vi "ScanPositionRange.vi"(8 "Target position":dbl, 9 "Start position":dbl, 10 "Velocity":dbl, 11 "Connection Cluster in":T1) -> (1 "Peak detected?":bool, 2 "output cluster":cluster{dbl[], dbl[]}, 3 "Connection Cluster out":T1)   [LabVIEW 2013]
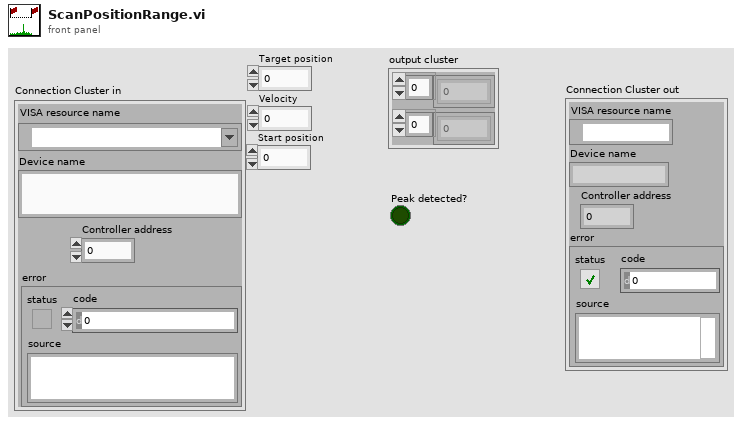
[diagram p1: front panel]
types:
  T1 = cluster{"VISA resource name":refnum<visa-resource-name>, "Device name":string, "Controller address":i32, "error":errorcluster}
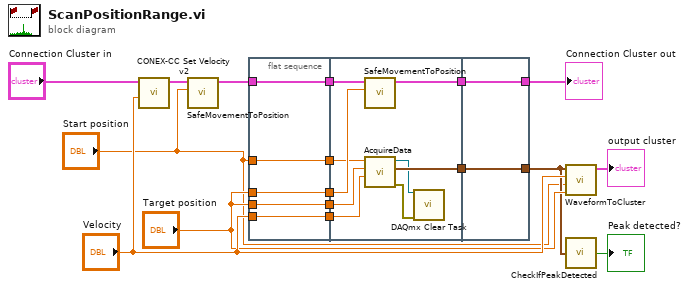
[diagram p0: block diagram]
diagram:
  n1 = call <userlib>:"CONEX-CC Set Velocity v2.vi"("Velocity"="Velocity", "Connection Cluster in"="Connection Cluster in") -> ("Connection Cluster out"=w14:T1)  [unwired: 9 in]
  n2 = call "SafeMovementToPosition.vi"("Target position"="Start position", "Connection Cluster in"=w14) -> ("Connection Cluster out"=w17:T1)  [unwired: 9 in]
  n3 = flat-sequence {
    tunnel: "Velocity" -> [w18]
    tunnel: "Target position" -> [w19]
    tunnel: "Start position" -> [w20]
    tunnel: "Target position" -> [w21]
    tunnel: w17 -> [w22]
    tunnel: [w22] -> w11
    tunnel: [w21] -> w10
    tunnel: [w20] -> w9
    tunnel: [w19] -> w8
    tunnel: [w18] -> w7
    tunnel: w11 -> [w31]
    tunnel: w10 -> [w28]
    tunnel: w9 -> [w27]
    tunnel: w8 -> [w26]
    tunnel: w7 -> [w25]
    tunnel: [w30] -> w6
    tunnel: [w29] -> w5
    tunnel: [w32] -> w3
    tunnel: [w33] -> w16
    tunnel: w6 -> [w33]
    tunnel: w5 -> [w32]
    frame #0 {
    }
    frame #1 {
      n4 = call "SafeMovementToPosition.vi"("Target position"=w28, "Connection Cluster in"=w31) -> ("Connection Cluster out"=w30:T1)  [unwired: 9 in]
      n5 = call "AcquireData.vi"("Velocity"=w25, "Target position"=w26, "Start position"=w27) -> ("error out"=w23:errorcluster, "data"=w29:waveform(dbl), "task out"=w24:refnum<k21>)  [unwired: 6 in]
      n6 = call <vilib>:"DAQmx Clear Task.vi"("task in"=w24, "error in"=w23) -> ()  [unwired: 13 in, 1 out]
    }
    frame #2 {
    }
  }
  n7 = call "WaveformToCluster.vi"("Target Position"="Target position", "Start Position"="Start position", "Velocity"="Velocity", "waveform"=w3) -> ("output cluster"=→"output cluster":cluster{dbl[], dbl[]})  [unwired: 7 in]
  n8 = call "CheckIfPeakDetected.vi"("data"=w3) -> ("Peak detected?"=→"Peak detected?":bool)
  "Connection Cluster out" <- w16
